vi "Actor Core.vi"(8 "error in":errorcluster, 11 "Form Window in":refnum<class "Form Window.lvclass">) -> (0 "error out":errorcluster, 3 "Actor out":refnum<class "Actor.lvclass">)   [LabVIEW 2020, in "Panel Form Controller.lvlib" / "Form Window.lvclass"]
doc: "The user interface for this panel.\n\n----\nPlease see the following web address for additional documentation and tutorial information:\nhttp://www.mooregoodideas.com/mgi-panel-manager/\n\nAuthor: Derek Trepanier\n\nCopyright (c) 2018, Moore Good Ideas, Inc.\n\nAll rights reserved.\n\nRedistribution and use in source and binary forms, with or without modification, are permitted provided that the following conditions are met:\n\n * Redistributions of source code must retain the above copyright notice, this list of conditions and the following disclaimer.\n * Redistributions in binary form must reproduce the above copyright notice, this list of conditions and the following disclaimer in the documentation and/or other materials provided with the distribution.\n * Neither the name of Moore Good Ideas, Inc. nor the names of its contributors may be used to endorse or promote products derived from this software without specific prior written permission.\n\nTHIS SOFTWARE IS PROVIDED BY THE COPYRIGHT HOLDERS AND CONTRIBUTORS \"AS IS\" AND ANY EXPRESS OR IMPLIED WARRANTIES, INCLUDING, BUT NOT LIMITED TO, THE IMPLIED WARRANTIES OF MERCHANTABILITY AND FITNESS FOR A PARTICULAR PURPOSE ARE DISCLAIMED. IN NO EVENT SHALL THE COPYRIGHT OWNER OR CONTRIBUTORS BE LIABLE FOR ANY DIRECT, INDIRECT, INCIDENTAL, SPECIAL, EXEMPLARY, OR CONSEQUENTIAL DAMAGES (INCLUDING, BUT NOT LIMITED TO, PROCUREMENT OF SUBSTITUTE GOODS OR SERVICES; LOSS OF USE, DATA, OR PROFITS; OR BUSINESS INTERRUPTION) HOWEVER CAUSED AND ON ANY THEORY OF LIABILITY, WHETHER IN CONTRACT, STRICT LIABILITY, OR TORT (INCLUDING NEGLIGENCE OR OTHERWISE) ARISING IN ANY WAY OUT OF THE USE OF THIS SOFTWARE, EVEN IF ADVISED OF THE POSSIBILITY OF SUCH DAMAGE."
uses:
  Form Window.lvclass
  C:/Users/User/Desktop/Raman Program/Database OOP/source/Forms AF/Form Controller/Panel Form Controller.lvclass
  <vilib>/ActorFramework/Actor/Actor.lvclass
  Form Controller/Panel Form Controller.lvclass/Panel Form Controller.ctl
  Controller Configuration/Panel Form Controller Configuration.lvclass/Panel Form Controller Configuration.ctl
  Controller Configuration/Panel Form Controller Configuration.lvclass
  Database OOP/Table Libraries/Basic Form/Basic Form.lvclass
  Form Controller/Panel Form Controller.lvclass
panel:
  in  "Add":bool
  in  "Primary Key":u16(ring)
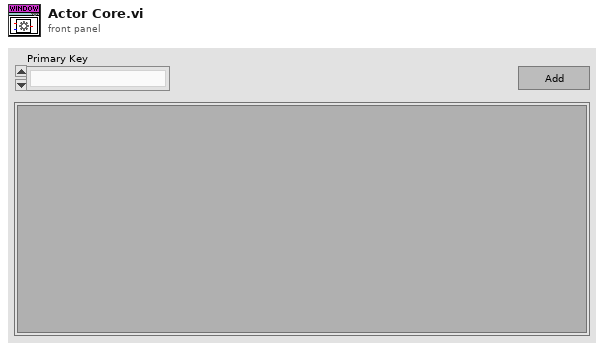
[diagram p1: front panel]
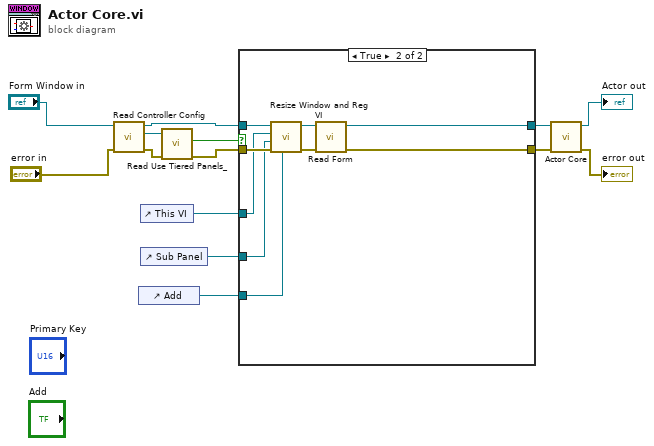
[diagram p0: block diagram]
diagram:
  n1 = call "Read Controller Config.vi"("error in (no error)"="error in", "Panel Form Controller in"="Form Window in") -> ("error out"=w7:errorcluster, "Controller Config"=w8:refnum<class "Panel Form Controller Configuration.lvclass">, "Panel Form Controller out"=w5:refnum<class "Form Window.lvclass">)  [unwired: 7 in]
  n2 = control-ref of="Add"() -> (w1:refnum<vi>)
  n3 = control-ref of="This VI"() -> (w3:refnum<vi>)
  n4 = control-ref of="Sub Panel"() -> (w2:refnum<vi>)
  n5 = call "Read Use Tiered Panels_.vi"("error in (no error)"=w7, "Panel Form Controller Configuration in"=w8) -> ("error out"=w4:errorcluster, "Use Tiered Panels?"=w6:bool)  [unwired: 7 in, 1 out]
  n6 = case shown="True" w6 {
    tunnel: [w16 w25] -> w11
    tunnel: [w15 w24] -> w10
    tunnel: w5 -> [w16 w23]
    tunnel: w4 -> [w15 w21]
    tunnel: w3 -> [_ w17]
    tunnel: w2 -> [_ w19]
    tunnel: w1 -> [_ w18]
    frame False {
    }
    frame True {
      n7 = call "Resize Window and Reg VI.vi"("Add Button Refnum"=w18, "error in (no error)"=w21, "Sub Panel Refnum"=w19, "Actor Core Refnum"=w17, "Form Window in"=w23) -> ("error out"=w20:errorcluster, "Form Window out"=w22:refnum<class "Form Window.lvclass">)  [unwired: 5 in]
      n8 = call "Read Form.vi"("error in (no error)"=w20, "Panel Form Controller in"=w22) -> ("error out"=w24:errorcluster, "Panel Form Controller out"=w25:refnum<class "Form Window.lvclass">)  [unwired: 7 in, 1 out]
    }
  }
  n9 = call-parent "Actor Core.vi"("error in"=w10, "Panel Form Controller in"=w11) -> ("error out"=→"error out":errorcluster, "Actor out"=→"Actor out":refnum<class "Actor.lvclass">)  [unwired: 8 in]
